vi "Send Write Record(sec).vi"(7 "Message Priority (Normal)":T2=enum."Normal", 8 "error in (no error)":errorcluster, 10 "Record":T1, 11 "Message Enqueuer":refnum<class "Message Enqueuer.lvclass">) -> (0 "error out":errorcluster, 3 "Message Enqueuer out":refnum<class "Message Enqueuer.lvclass">)   [LabVIEW 2019, in "Configuration Database Actor.lvlib" / "Write Record(sec) Msg.lvclass"]
doc: "This VI sends the message to an actor."
uses:
  Write Record(sec) Msg.lvclass
  <vilib>/ActorFramework/Message Enqueuer/Message Enqueuer.lvclass
  C:/Program Files (x86)/National Instruments/LabVIEW 2019/vi.lib/ActorFramework/Message/Message.lvclass
  <vilib>/ActorFramework/Message Enqueuer/Message Priority.ctl
  Configuration Database Actor/Record -Cluster.ctl
  Configuration Database Actor/Configuration Database Actor.lvclass
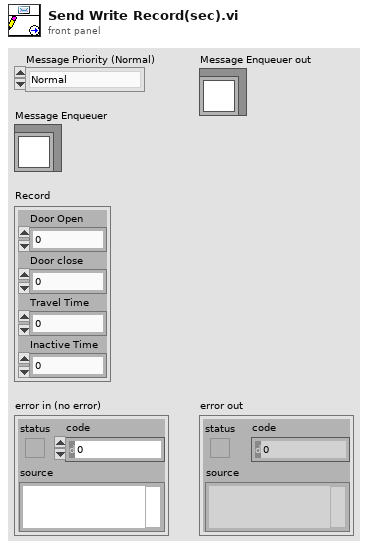
[diagram p1: front panel]
types:
  T1 = typedef "Configuration Database Actor.lvlib/Configuration Database Actor.lvclass/Record -Cluster.ctl" = cluster{"Door Open":dbl, "Door close":dbl, "Travel Time":dbl, "Inactive Time":dbl}
  T2 = typedef "Actor Framework.lvlib/Message Enqueuer.lvclass/Message Priority.ctl" = enum16{"Low", "Normal", "High"}
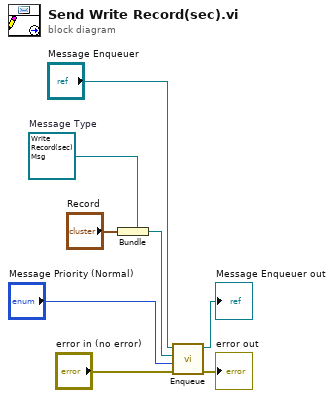
[diagram p0: block diagram]
diagram:
  w5 = refnum<class "Write Record(sec) Msg.lvclass"> refnum  # Message Type
  n1 = Bundle(cluster=w5, "Record") -> (w4:refnum<class "Write Record(sec) Msg.lvclass">)
  n2 = call <vilib>:"Enqueue.vi"("error in (no error)"="error in (no error)", "Message Priority (Normal)"="Message Priority (Normal)", "Message"=w4, "Message Enqueuer in"="Message Enqueuer") -> ("error out"=→"error out":errorcluster, "Message Enqueuer out"=→"Message Enqueuer out":refnum<class "Message Enqueuer.lvclass">)  [unwired: 6 in]
